vi "PLC初始化.vi"(8 "错误输入（无错误）":errorcluster, 11 "ipAddress":string) -> (0 "错误输出":errorcluster, 1 "IsSuccess":bool, 3 "引用输出":refnum<k24>)   [LabVIEW 2021]
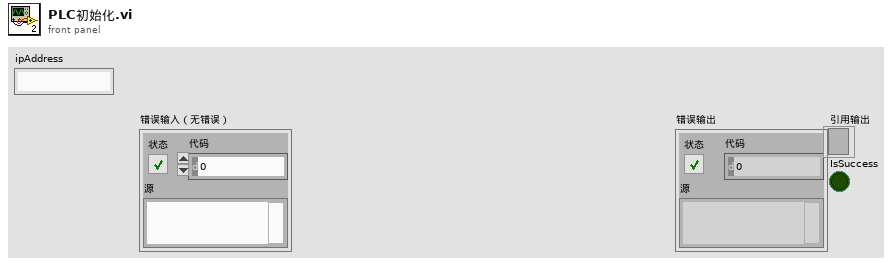
[diagram p1: front panel]
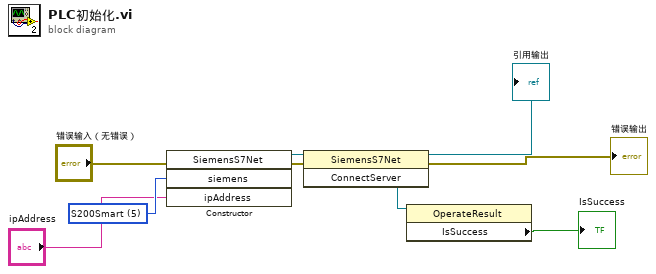
[diagram p0: block diagram]
diagram:
  w6 = 5 items=["S1200"=1, "S300"=2, "S400"=3, "S1500"=4, "S200Smart"=5, "S200"=6] ("siemens")
  n1 = constructor class="SiemensS7Net"(error in="错误输入（无错误）", "siemens"=w6, "ipAddress"="ipAddress") -> (reference out=w8:refnum<k24>, error out=w9:errorcluster)  [unwired: 2 in, 3 out]
  n2 = invoke class="SiemensS7Net" method="ConnectServer"(reference=w8, error in=w9) -> (reference out=→"引用输出":refnum<k24>, error out=→"错误输出":errorcluster, "ConnectServer"=w7:refnum<k24>)  [unwired: 1 in]
  n3 = property class="OperateResult"(reference=w7) -> ("IsSuccess"=→"IsSuccess":bool)  [unwired: 1 in, 2 out]
